vi "TP Buffer Convert Connection Info to CAN Frame.vi"(0 "Connection Cluster":T3, 11 "error in (no error)":errorcluster) -> (4 "CAN frame":T1 {"payload" format="%x"; "timestamp" format="%<%.7X\n%x>T"; "type" items=["CAN Data"=0, "CAN Remote"=1, "CAN Bus Error"=2, "J1939 Data"=192, "Delay"=224, "Log Trigger"=225, "Start Trigger"=226]; "identifier" format="%x"}, 15 "error out":errorcluster)   [LabVIEW 2013, in "J1939.lvlib"]
uses:
  J1939.lvlib
  TP Buffer Connection Cluster.ctl
  <vilib>/xnet/xnet.llb/XNET Frame CAN.ctl
  <vilib>/xnet/xnet.llb/XNET Frame Type CAN.ctl
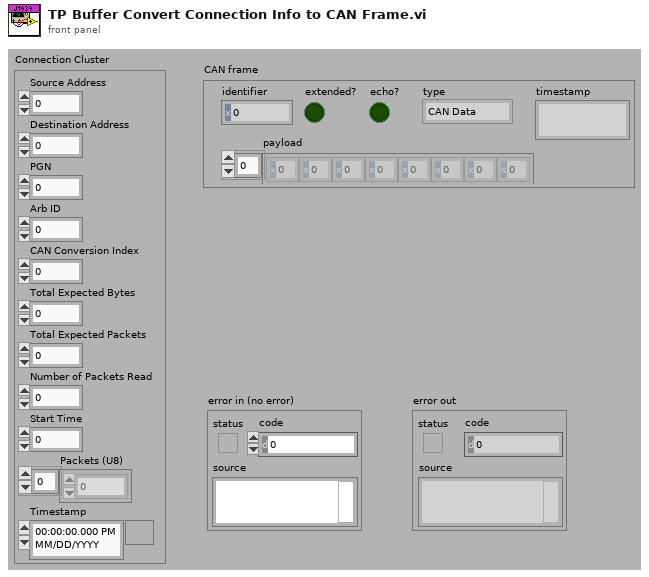
[diagram p1: front panel]
types:
  T1 = typedef "XNET Frame CAN.ctl" = cluster{"timestamp":timestamp, "payload":u8[], "identifier":u32, "type":T2, "extended?":bool, "echo?":bool}
  T2 = typedef "XNET Frame Type CAN.ctl" = u8
  T3 = typedef "J1939.lvlib/TP Buffer Connection Cluster.ctl" = cluster{"Source Address":u8, "Destination Address":u8, "PGN":u32, "Arb ID":u32, "CAN Conversion Index":u32, "Total Expected Bytes":u16, "Total Expected Packets":u8, "Number of Packets Read":u8, "Start Time":u32, "Packets (U8)":u8[], "Timestamp":timestamp}
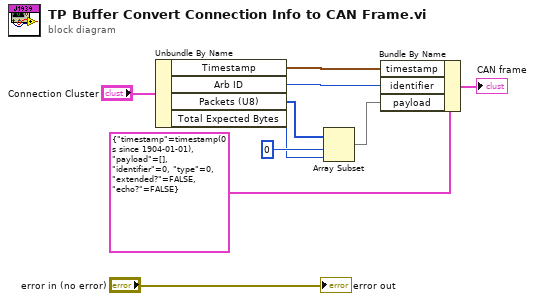
[diagram p0: block diagram]
diagram:
  n1 = Unbundle By Name("Connection Cluster") -> ("Timestamp"=w9:timestamp, "Arb ID"=w8:u32, "Packets (U8)"=w4:u8[], "Total Expected Bytes"=w5:u16)
  n2 = Array Subset(array=w4, index=0, length=w5) -> (w3:u8[])
  n3 = Bundle By Name(cluster=T1 {"timestamp"=timestamp(0 s since 1904-01-01), "payload"=[], "identifier"=0, "type"=0, "extended?"=FALSE, "echo?"=FALSE} ("CAN frame"), "timestamp"=w9, "identifier"=w8, "payload"=w3) -> (→"CAN frame":T1)
  "error out" <- "error in (no error)"
